vi "Station.Initialize.vi"(8 "error in (no error)":errorcluster, 11 "state variables in":T1) -> (0 "error out":errorcluster, 3 "state variables out":T1)   [LabVIEW 2015, in "Stations.Overview.lvlib"]
uses:
  Stations.Overview.lvlib
  Types/Overview.StateVariables.ctl
  Types/Overview.Channels.ctl
  <vilib>/NI Veristand/Execution/Workspace/SystemStateEventRef.ctl
  <vilib>/NI Veristand/Execution/Workspace/Target State Info.ctl
  <vilib>/NI Veristand/Execution/Workspace/Target State.ctl
  <vilib>/NI Veristand/Execution/Workspace/WorkspaceAPI.ctl
  NationalInstruments.VeriStand.ClientAPI
  Execution GUI/Types/Execute.UserEventRefs.ctl
  <vilib>/NI Veristand/Execution/Workspace/SystemStateRegEventRef.ctl
  <vilib>/NI Veristand/Execution/WaveformStreaming/Waveform Data Watcher Event Data (DBL).ctl
  <vilib>/NI Veristand/Execution/WaveformStreaming/WaveformStreamSpecification.ctl
  <vilib>/Utility/miscctls.llb/LVRowAndColumnTypeDef.ctl
  <vilib>/NI/AMC/Queue Registry.vi
  <vilib>/NI/AMC/AMC.lvlib
  <vilib>/NI Veristand/Execution/Workspace/NI_VS Workspace ExecutionAPI.lvlib
  Execution GUI/Station.Execution.lvlib
  <vilib>/NI Veristand/Execution/WaveformStreaming/NI_VS Waveform Streaming Interface.lvlib
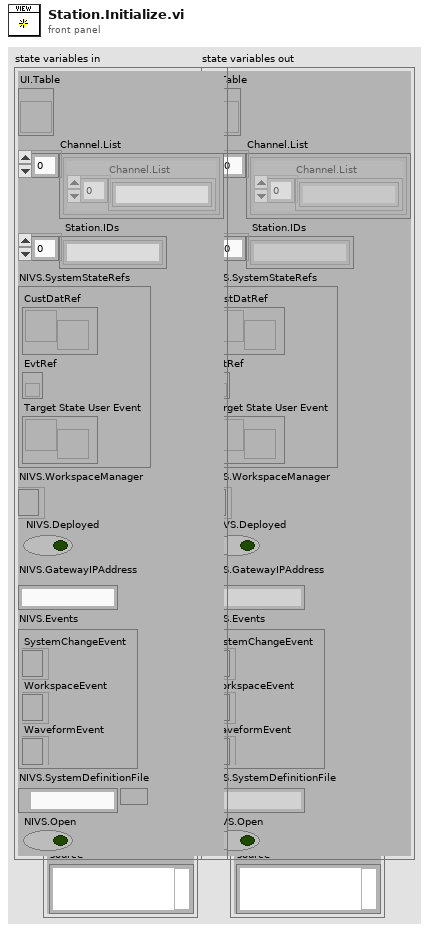
[diagram p1: front panel]
types:
  T1 = typedef "Stations.Overview.lvlib/Overview.StateVariables.ctl" = cluster{"UI.Table":refnum<vi>, "Channel.List":T2[], "Station.IDs":string[], "NIVS.SystemStateRefs":T3, "NIVS.WorkspaceManager":T4, "NIVS.Deployed":bool, "NIVS.GatewayIPAddress":string, "NIVS.Events":T5, "NIVS.SystemDefinitionFile":path, "NIVS.Open":bool}
  T2 = typedef "Stations.Overview.lvlib/Overview.Channels.ctl" = cluster{"Channel.List":string[]}
  T3 = typedef "NI_VS Workspace ExecutionAPI.lvlib/SystemStateEventRef.ctl" = cluster{"CustDatRef":refnum<user-event>, "EvtRef":refnum<k27>, "Target State User Event":refnum<user-event>}
  T4 = typedef "NI_VS Workspace ExecutionAPI.lvlib/WorkspaceAPI.ctl" = refnum<k24>
  T5 = typedef "Station.Execution.lvlib/Execute.UserEventRefs.ctl" = cluster{"SystemChangeEvent":T6, "WorkspaceEvent":refnum<event-registration>, "WaveformEvent":refnum<event-registration>}
  T6 = typedef "NI_VS Workspace ExecutionAPI.lvlib/SystemStateRegEventRef.ctl" = refnum<event-registration>
  T7 = typedef "LVRowAndColumnTypeDef.ctl" = cluster{"Row":i32, "Column":i32}
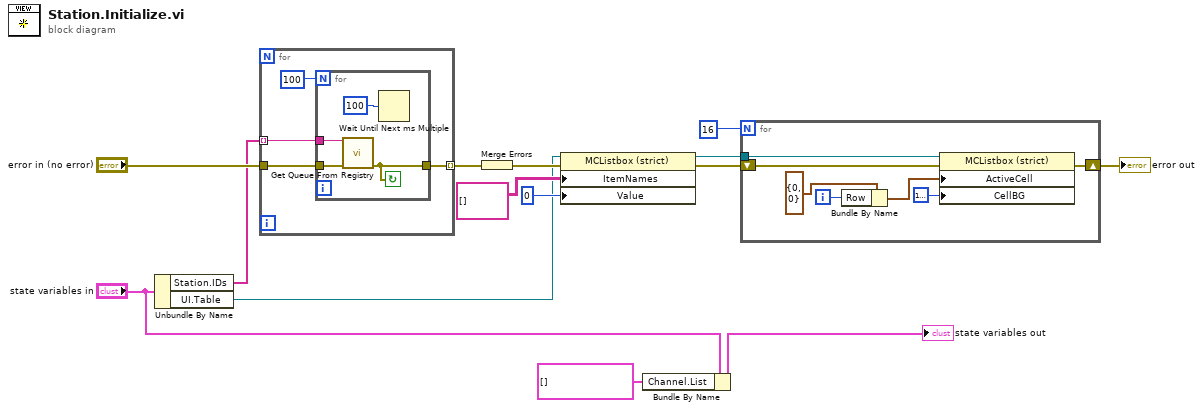
[diagram p0: block diagram]
diagram:
  n1 = Unbundle By Name("state variables in") -> ("Station.IDs"=w10:string[], "UI.Table"=w4:refnum<vi>)
  n2 = for {
    tunnel: w10 -> [w18] mode=indexing
    tunnel: [w16] -> w11 mode=indexing
    tunnel: "error in (no error)" -> [w15]
    n3 = for {
      N: 100 -> [_]
      tunnel: w18 -> [w22]
      tunnel: [w20] -> w16
      tunnel: w15 -> [w19]
      stop <- w20 continue-if-true
      n4 = call <vilib>:"Get Queue From Registry.vi"("name"=w22, "error in"=w19) -> ("error out"=w20:errorcluster)  [unwired: 12 in, 1 out]
      n5 = Wait Until Next ms Multiple(millisecond multiple=u32 100) -> ()  [unwired: 1 out]
    }
  }
  n6 = Merge Errors(w11) -> (w13:errorcluster)
  n7 = property class="MCListbox (strict)"(reference=w4, error in=w13, "ItemNames"=string[][] [] ("Item Names"), "Value"=0) -> (reference out=w7:refnum<vi>, error out=w8:errorcluster)
  n8 = Bundle By Name(cluster="state variables in", "Channel.List"=T2[] []) -> (→"state variables out":T1)
  n9 = for {
    N: 16 -> [_]
    tunnel: w7 -> [w29]
    shift-right: [w27] -> w14
    shift-left: w8 -> [w28]
    i -> [w23]
    n10 = Bundle By Name(cluster=T7 {"Row"=0, "Column"=0} ("Active Cell:Active Cell"), "Row"=w23) -> (w24:T7)
    n11 = property class="MCListbox (strict)"(reference=w29, error in=w28, "ActiveCell"=w24, "CellBG"=u32 16777216) -> (error out=w27:errorcluster)  [unwired: 1 out]
  }
  "error out" <- w14
